vi "Ejemplo_ReporteHTML.vi"() -> ()   [LabVIEW 2025]
uses:
  <vilib>/Utility/NIReport.llb/Report Type.ctl
  <vilib>/Utility/NIReport.llb/Append Report Text (str wrap).vi
  <vilib>/printing/OpenHTMLReport.llb/Open HTML Report in Browser (Refnum).vi
  <vilib>/Utility/NIReport.llb/NI_report.lvclass
  <vilib>/Utility/NIReport.llb/NI_ReportGenerationCore.lvlib
panel:
  in  "Cuerpo 1":string="\n\n<div align=\"center\" style=\"font-family: Arial, sans-serif;\">\n    \n    <!-- Encabezado con Logos usando una Tabla para alinear Izquierda, Centro y Derecha -->\n    <table width=\"100%\" border=\"0\" style=\"margin-bottom: 20px;\">\n        <tr>\n            <!-- Logo Izquierdo (IPN) -->\n            <td width=\"20%\" align=\"center\" valign=\"middle\">\n                <img src=\"file:///C:/Users/julio/OneDrive%20-%20Instituto%20Politecnico%20Nacional/Documents/Implementacion_Virtual/LOGOIPN.png\" width=\"350\" alt=\"Logo IPN\">\n            </td>\n            \n            <!-- Títulos Centrales -->\n            <td width=\"60%\" align=\"center\" valign=\"middle\">\n                <h1 style=\"font-size: 30px; font-weight: bold; margin: 0; color: #333333;\">INSTITUTO POLIT&Eacute;CNICO NACIONAL</h1>\n                <h2 style=\"font-size: 24px; margin: 5px 0 0 0; color: #444444;\">UNIDAD PROFESIONAL INTERDISCIPLINARIA DE INGENIER&Iacute;A CAMPUS ZACATECAS (UPIIZ)</h2>\n            </td>\n            \n            <!-- Logo Derecho (UPIIZ) -->\n            <td width=\"20%\" align=\"center\" valign=\"middle\">\n                <img src=\"file:///C:/Users/julio/OneDrive%20-%20Instituto%20Politecnico%20Nacional/Documents/Implementacion_Virtual/UPIIZ1.png\" width=\"200\" alt=\"Logo UPIIZ\">\n            </td>\n        </tr>\n    </table>\n    \n    <br>\n    \n    <h3 style=\"font-size: 22px;\">Programa Acad&eacute;mico:</h3>\n    <p style=\"font-size: 20px;\">Ingenier&iacute;a en Mecatr&oacute;nica</p>\n    \n    <br>\n    \n    <h3 style=\"font-size: 22px;\">Unidad de Aprendizaje:</h3>\n    <p style=\"font-size: 20px;\">Implementacion virtual aplicada  avanzada</p>\n    \n    \n    <h3 style=\"font-size: 22px;\">T&iacute;tulo del Trabajo / Pr&aacute;ctica:</h3>\n    <p style=\"font-size: 20px;\"><b style=\"color: #6A1B31;\">Unidad 02 Pr&aacute;ctica 02.<br>Control de Temperatura mediante L&oacute;gica Difusa (Fuzzy).</b></p>\n    \n    <br><br><br>\n    \n    <h3 style=\"font-size: 22px;\">Presentan:</h3>\n    <p style=\"font-size: 20px;\">\n        Diego Adair Delgado Hern&aacute;ndez. 4MM3.<br>\n        Julio Cesar Nu&ntilde;ez Qui&ntilde;ones. 4MM3.\n    </p>\n    \n    <br><br>\n    \n    <h3 style=\"font-size: 22px;\">Profesor:</h3>\n    <p style=\"font-size: 20px;\">Ramon jaramillo</p>\n    \n    <br><br><br>\n    \n    <p style=\"font-size: 20px;\">Zacatecas, Zac., a 03 de Junio de 2026</p>\n</div>\n<!-- SALTO PARA LA NUEVA SECCIÓN -->\n<br><br><hr><br><br>\n<div align=\"justify\" style=\"font-family: Arial, sans-serif; font-size: 16px; line-height: 1.6; margin-left: 20px; margin-right: 20px;\">\n    \n    <h2 style=\"text-align: left; color: #333333; font-size: 22px;\">Introducci&oacute;n</h2>\n    \n    El control de temperatura es un desaf&iacute;o cl&aacute;sico en la ingenier&iacute;a debido a las no linealidades y la inercia t&eacute;rmica que presentan los sistemas de calentamiento. A diferencia del control cl&aacute;sico (como el PID) que requiere un modelo matem&aacute;tico exacto de la planta, el <strong style=\"color: #6A1B31;\">Control L&oacute;gico Difuso (Fuzzy Logic Control)</strong> ofrece una alternativa robusta basada en el razonamiento humano emp&iacute;rico.</p>\n    <p>La l&oacute;gica difusa permite mapear variables de entrada, como el error de temperatura respecto al <i>Set Point</i>, en conjuntos difusos (por ejemplo: \"Fr&iacute;o\", \"Adecuado\", \"Caliente\") para tomar decisiones de control mediante reglas ling&uuml;&iacute;sticas del tipo <i>IF-THEN</i>. En esta pr&aacute;ctica se utiliza <strong style=\"color: #6A1B31;\">LabVIEW</strong> junto con su m&oacute;dulo de l&oacute;gica difusa para dise&ntilde;ar e implementar un controlador tipo SISO (<i>Single-Input Single-Output</i>) u otros modelos. A trav&eacute;s de un DAQ Assistant se adquiere la temperatura real del sistema para calcular el error; posteriormente, el controlador difuso procesa dicho error para establecer la se&ntilde;al de control adecuada, la cual suele determinar el ciclo de trabajo (<i>Duty Cycle</i>) del actuador. Este m&eacute;todo permite estabilizar la temperatura de manera suave, reduciendo sobreimpulsos y oscilaciones de forma muy eficiente sin necesidad de m&eacute;todos de sintonizaci&oacute;n complejos.\n    <br>\n    \n    <h2 style=\"text-align: left; color: #333333; font-size: 22px;\">Desarrollo</h2>\n    \n    La implementaci&oacute;n de nuestro sistema de control de temperatura se llev&oacute; a cabo estructurando el diagrama de bloques en distintas etapas l&oacute;gicas, lo cual permite un flujo de datos limpio y f&aacute;cil de depurar. A continuaci&oacute;n, se detalla paso a paso el funcionamiento del sistema dise&ntilde;ado en LabVIEW:\n    \n    <ul style=\"margin-bottom: 20px;\">\n        <li style=\"margin-bottom: 10px;\"><strong>1. Adquisici&oacute;n y Acondicionamiento de Datos:</strong> El proceso inicia con el bloque <i>DAQ Assistant</i>, el cual se encarga de leer la se&ntilde;al anal&oacute;gica proveniente del sensor de temperatura f&iacute;sico acoplado a nuestra planta. Esta se&ntilde;al cruda pasa por una etapa de acondicionamiento (escalamiento matem&aacute;tico) para convertir el voltaje medido en una lectura real de temperatura (Temp) en grados cent&iacute;grados.</li>\n        \n        <li style=\"margin-bottom: 10px;\"><strong>2. C&aacute;lculo del Error:</strong> La base de cualquier control en lazo cerrado es conocer qu&eacute; tan lejos estamos de nuestra meta. La variable <i>Temp</i> se resta directamente del <i>Set point</i> (nuestra temperatura deseada, ingresada desde el panel frontal). El resultado de esta sustracci&oacute;n genera la se&ntilde;al de <i>Error</i>, la cual es cr&iacute;tica para el controlador.</li>\n        \n        <li style=\"margin-bottom: 10px;\"><strong>3. Etapa de L&oacute;gica Difusa (Bloque SISO):</strong> El <i>Error</i> (junto con la lectura de temperatura, dependiendo de la arquitectura) entra al n&uacute;cleo del sistema: el bloque controlador SISO de L&oacute;gica Difusa. Internamente, este bloque procesa las reglas dise&ntilde;adas en el <i>Fuzzy System Designer</i>. En este espacio, valores num&eacute;ricos fr&iacute;os se traducen a grados de pertenencia (ej. \"Muy Lejos\", \"Cerca\", \"Caliente\"). Mediante reglas tipo <i>IF-THEN</i> (Ej. \"SI el error es Positivo Grande, ENTONCES encender al m&aacute;ximo\"), el sistema infiere qu&eacute; porcentaje de energ&iacute;a se requiere, entregando en su salida un valor n&iacute;tido que representa el Ciclo de Trabajo (<i>Duty Cycle</i>) ideal.</li>\n        \n        <li style=\"margin-bottom: 10px;\"><strong>4. Generaci&oacute;n de la se&ntilde;al de control (PWM):</strong> El valor de salida del bloque difuso es un porcentaje (0 a 100). Para traducir este porcentaje en algo que un actuador f&iacute;sico (como un rel&eacute; de estado s&oacute;lido o resistencia calentadora) pueda entender, usamos operaciones matem&aacute;ticas. El <i>Duty</i> se divide entre 100 y se multiplica por el per&iacute;odo de operaci&oacute;n de nuestro sistema (aproximadamente 16.66 milisegundos, que corresponde a un semiciclo de la red el&eacute;ctrica a 60 Hz). Esto nos da como resultado el <i>High Time</i> (tiempo en alto). Al restarle el tiempo en alto al per&iacute;odo total de 16.666 ms, obtenemos el <i>Low Time</i> (tiempo en bajo). Estas dos variables son las que finalmente dictan el pulso de conmutaci&oacute;n del calentador.</li>\n        \n        <li style=\"margin-bottom: 10px;\"><strong>5. Interfaz de Usuario e Indicadores Gr&aacute;ficos:</strong> De forma paralela, variables como el Set Point y la Temperatura actual se agrupan mediante un <i>Merge Signals</i> y se env&iacute;an a un <i>Waveform Chart</i>. Esto nos permite visualizar en tiempo real c&oacute;mo la temperatura de la planta sube suavemente hasta estabilizarse justo en el Set point, demostrando emp&iacute;ricamente la capacidad de la l&oacute;gica difusa para evitar los t&iacute;picos sobreimpulsos (overshoots) de los controladores cl&aacute;sicos mal sintonizados.</li>\n    </ul>\n    En las siguientes figuras se evidencia el Panel Frontal del VI, as&iacute; como el Diagrama de Bloques completo y las superficies de control configuradas en el dise&ntilde;ador difuso.</p>\n    <br><br>\n    \n    <!-- SECCIÓN DE IMÁGENES -->\n    <h3 style=\"text-align: center; color: #333333;\">1.- Control fuzzy</h3>\n    <div style=\"text-align: center; margin-bottom: 20px;\">\n        <img src=\"file:///C:/Users/julio/OneDrive%20-%20Instituto%20Politecnico%20Nacional/Documents/Implementacion_Virtual/IMA1.png\" style=\"max-width: 100%; border: 1px solid #cccccc;\" alt=\"IMA1\">\n    </div>\n    \n    <br><br>\n    \n    <h3 style=\"text-align: center; color: #333333;\">2.- PWM</h3>\n    <div style=\"text-align: center; margin-bottom: 20px;\">\n        <img src=\"file:///C:/Users/julio/OneDrive%20-%20Instituto%20Politecnico%20Nacional/Documents/Implementacion_Virtual/IMA2.png\" style=\"max-width: 100%; border: 1px solid #cccccc;\" alt=\"IMA2\">\n    </div>\n    \n    <br><br>\n    \n    <h3 style=\"text-align: center; color: #333333;\">3.- EXCEL</h3>\n    <div style=\"text-align: center; margin-bottom: 20px;\">\n        <img src=\"file:///C:/Users/julio/OneDrive%20-%20Instituto%20Politecnico%20Nacional/Documents/Implementacion_Virtual/IMA3.png\" style=\"max-width: 100%; border: 1px solid #cccccc;\" alt=\"IMA3\">\n    </div>\n    \n    <br><br>\n    \n    <h3 style=\"text-align: center; color: #333333;\">4.- Datos obtenidos de LabVIEW</h3>\n    <div style=\"text-align: center; margin-bottom: 20px;\">\n        <img src=\"file:///C:/Users/julio/OneDrive%20-%20Instituto%20Politecnico%20Nacional/Documents/Implementacion_Virtual/IMA5.png\" style=\"max-width: 100%; border: 1px solid #cccccc;\" alt=\"IMA5 - Datos LabVIEW\">\n    </div>\n\n    <br><br>\n    \n    <h3 style=\"text-align: center; color: #333333;\">5.- Panel Frontal</h3>\n    <div style=\"text-align: center; margin-bottom: 20px;\">\n        <img src=\"file:///C:/Users/julio/OneDrive%20-%20Instituto%20Politecnico%20Nacional/Documents/Implementacion_Virtual/IMA6.png\" style=\"max-width: 100%; border: 1px solid #cccccc;\" alt=\"IMA6 - Panel Frontal\">\n    </div>\n    \n</div>\n\n\n\n<!-- CÓDIGO HTML PARA LA CONCLUSIÓN -->\n<br><br><hr><br><br>\n\n<div align=\"justify\" style=\"font-family: Arial, sans-serif; font-size: 16px; line-height: 1.6; margin-left: 20px; margin-right: 20px;\">\n    \n    <h2 style=\"text-align: left; color: #333333; font-size: 22px;\">Conclusi&oacute;n</h2>\n    \n    <p>La implementaci&oacute;n de un controlador de temperatura utilizando l&oacute;gica difusa en LabVIEW demostr&oacute; ser una alternativa altamente eficaz, pr&aacute;ctica y robusta frente a los m&eacute;todos de control cl&aacute;sico, como el PID tradicional. A lo largo de esta pr&aacute;ctica, se comprob&oacute; que no es estrictamente necesario contar con un modelo matem&aacute;tico complejo y exacto de la planta t&eacute;rmica para lograr una estabilizaci&oacute;n adecuada. En su lugar, el conocimiento emp&iacute;rico sobre el comportamiento din&aacute;mico de la temperatura se logr&oacute; plasmar exitosamente a trav&eacute;s de la definici&oacute;n intuitiva de funciones de pertenencia y reglas ling&uuml;&iacute;sticas del tipo <i>IF-THEN</i>, utilizando la herramienta <i>Fuzzy System Designer</i>.</p>\n    \n    <p>La sintonizaci&oacute;n de este controlador destac&oacute; por su simplicidad, ya que el operador s&oacute;lo necesita ajustar l&oacute;gicamente c&oacute;mo reaccionar&iacute;a un humano ante los cambios (por ejemplo, si la temperatura est&aacute; muy fr&iacute;a, aplicar m&aacute;xima potencia; si est&aacute; cerca del valor deseado, reducir gradualmente el calor). Esta capacidad de adaptaci&oacute;n natural convierte a la l&oacute;gica difusa en una herramienta invaluable para procesos industriales donde los par&aacute;metros f&iacute;sicos var&iacute;an con el tiempo o son dif&iacute;ciles de modelar, demostrando as&iacute; una notable flexibilidad y tolerancia ante perturbaciones externas.</p>\n\n    <p>Adem&aacute;s, la integraci&oacute;n del m&oacute;dulo SISO con el procesamiento matem&aacute;tico dise&ntilde;ado para generar la se&ntilde;al de modulaci&oacute;n por ancho de pulsos (PWM) evidenci&oacute; c&oacute;mo un razonamiento abstracto y difuso puede traducirse directamente en una acci&oacute;n f&iacute;sica de hardware precisa. Al transformar el <i>Duty Cycle</i> inferido por el sistema difuso en tiempos de encendido y apagado (<i>High/Low Time</i>), se consigui&oacute; gobernar el elemento calefactor de forma fluida y sin saltos abruptos de energ&iacute;a.</p>\n    \n    <p>Finalmente, los datos adquiridos y las gr&aacute;ficas proyectadas en el panel frontal reflejan con claridad el &eacute;xito del sistema. El controlador es capaz de guiar la temperatura de la planta hasta alcanzar el <i>Set Point</i> establecido de manera suave y sostenida. Al observar la gr&aacute;fica resultante, se aprecia c&oacute;mo se mitigan casi por completo los caracter&iacute;sticos sobreimpulsos (<i>overshoots</i>) prolongados y las oscilaciones estacionarias que suelen provocar ineficiencias energ&eacute;ticas o incluso da&ntilde;os en los materiales de sistemas puramente on/off o mal sintonizados. En resumen, LabVIEW nos brind&oacute; un entorno gr&aacute;fico de desarrollo integrado y vers&aacute;til que facilit&oacute; cada fase del proyecto: desde la adquisici&oacute;n limpia de la se&ntilde;al an&aacute;loga a trav&eacute;s del Asistente DAQ, pasando por la inferencia l&oacute;gica avanzada, hasta culminar en el acondicionamiento de potencia y el monitoreo virtual en tiempo real.</p>\n\n</div>\n"
  out "Archivo temporal HTML":path
  in  "Encabezado":string
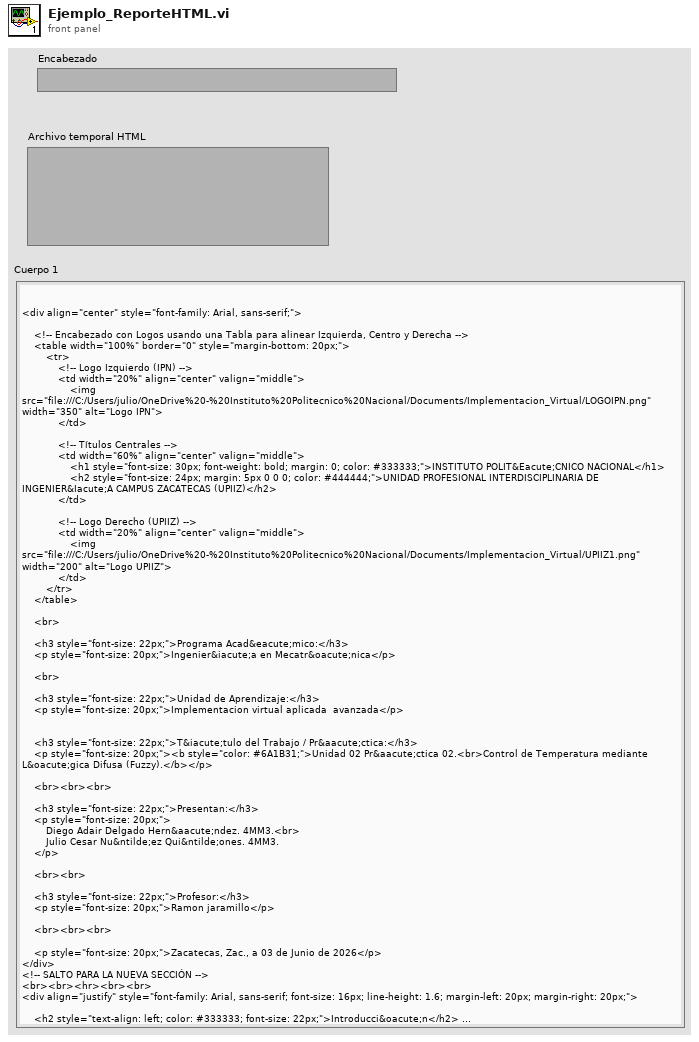
[diagram p1: front panel]
types:
  T1 = typedef "NI_ReportGenerationCore.lvlib/Report Type.ctl" = enum16{"HTML", "Word", "Excel"}
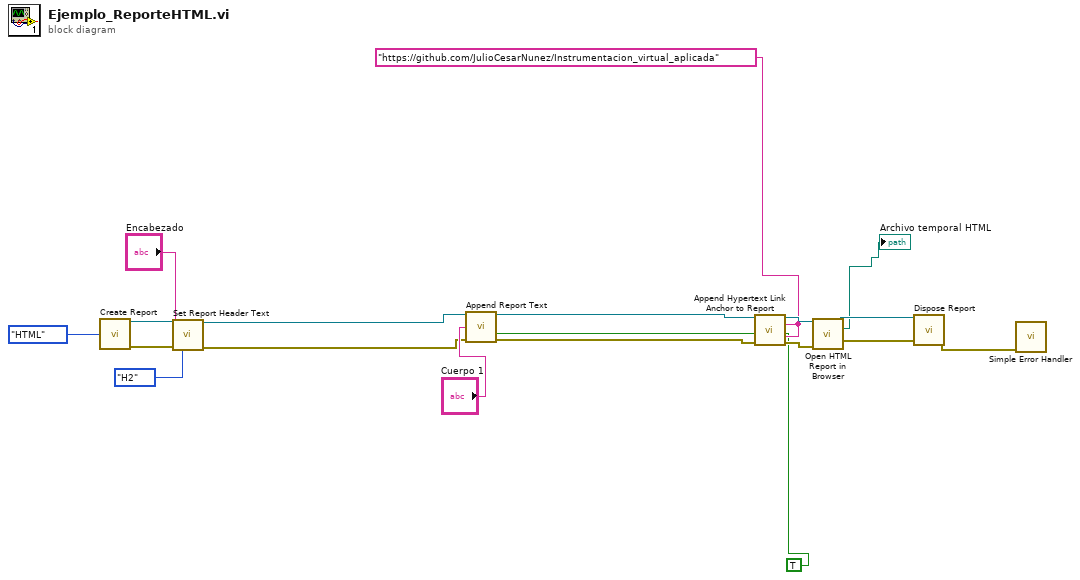
[diagram p0: block diagram]
diagram:
  w7 = "https://github.com/JulioCesarNunez/Instrumentacion_virtual_aplicada" ("URL of link - href")
  n1 = call <vilib>:"Create Report.vi"("report type"=Report_Type."HTML") -> ("report out"=w16:refnum<class "NI_report.lvclass">, "error out"=w15:errorcluster)  [unwired: 13 in]
  n2 = call-dynamic "Set Report Header Text.vi"("report in"=w16, "center header text"="Encabezado", "error in (no error)"=w15, "HTML header size"=enum16{"H1", "H2", "H3", "H4", "H5", "H6", "H7"}."H2") -> ("report out"=w2:refnum<class "NI_report.lvclass">, "error out"=w1:errorcluster)  [unwired: 10 in]
  n3 = call-poly <vilib>:"Append Report Text.vi"("report in"=w2, "text"="Cuerpo 1", "append on new line? (F)"=TRUE, "error in (no error)"=w1) -> ("report out"=w4:refnum<class "NI_report.lvclass">, "error out"=w3:errorcluster)  [unwired: 8 in, 2 out]
  n4 = call-dynamic "Append Hypertext Link Anchor to Report.vi"("report in"=w4, "URL of link - href"=w7, "link text"=w7, "error in (no error)"=w3) -> ("report out"=w10:refnum<class "NI_report.lvclass">, "error out"=w9:errorcluster)  [unwired: 8 in, 2 out]
  n5 = call-poly <vilib>:"Open HTML Report in Browser.vi"("report in"=w10, "error in (no error)"=w9) -> ("report out"=w13:refnum<class "NI_report.lvclass">, "temporary HTML file created"=→"Archivo temporal HTML":path, "error out"=w12:errorcluster)  [unwired: 11 in]
  n6 = call-dynamic "Dispose Report.vi"("report in"=w13, "error in (no error)"=w12) -> ("error out"=w11:errorcluster)  [unwired: 13 in]
  n7 = call <vilib>:"Simple Error Handler.vi"("error in (no error)"=w11) -> ()  [unwired: 4 in, 5 out]
